vi "F Dwf Digital Spi Write One.vi"(7 "vTX":u32, 8 "error in (no error)":errorcluster, 9 "cBits":i32, 10 "cDQ":i32, 11 "hdwf":i32) -> (0 "error out":errorcluster, 3 "function return":i32)   [LabVIEW 2021, in "Olasdwf.lvlib"]
doc: "DWFAPI int FDwfDigitalSpiWriteOne(HDWF hdwf, int cDQ, int cBits, unsigned int vTX);"
uses:
  Olasdwf.lvlib
  Windows/System32/dwf.dll
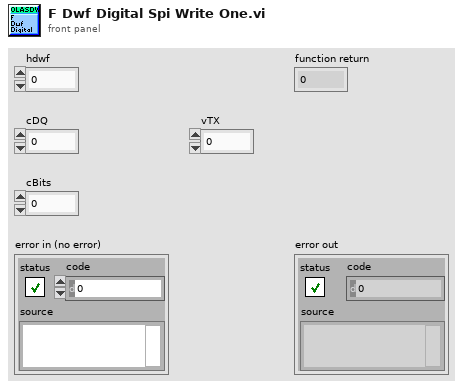
[diagram p1: front panel]
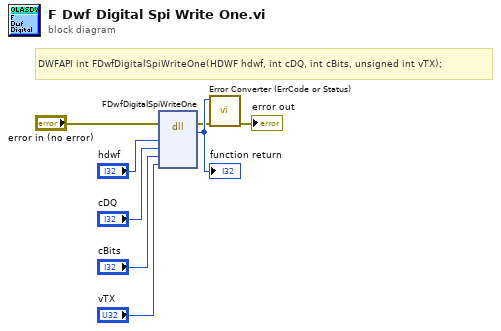
[diagram p0: block diagram]
diagram:
  # "DWFAPI int FDwfDigitalSpiWriteOne(HDWF hdwf, int cDQ, int cBits, unsigned int vTX);"
  n1 = dll-call lib="/Windows/System32/dwf.*" fn="FDwfDigitalSpiWriteOne"(error in="error in (no error)", "hdwf"="hdwf", "cDQ"="cDQ", "cBits"="cBits", "vTX"="vTX") -> (error out=w2:errorcluster, w8:i32)  [unwired: 6 in, 1 out]
  "function return" <- w8
  n2 = call "Error Converter (ErrCode or Status).vi"("error in (no error)"=w2, "error code"=w8) -> ("error out"=→"error out":errorcluster)  [unwired: 9 in]
